vi "add Device.vi"(8 "error in (no error)":errorcluster caption="Fehler (Eingang, kein Fehler)", 10 "Device.lvclass":refnum<class "Device.lvclass">, 11 "Setup Eingang":refnum<class "Setup.lvclass"> caption="DNL_LabVIEW Object in") -> (0 "error out":errorcluster caption="Fehler (Ausgang)", 3 "Setup Ausgang":refnum<class "Setup.lvclass"> caption="DNL_LabVIEW Object out")   [LabVIEW 2013, in "DatenKlassen.lvlib" / "Setup.lvclass"]
uses:
  Setup.lvclass
  Device/Device.lvclass
  Setup.lvclass/Setup.ctl
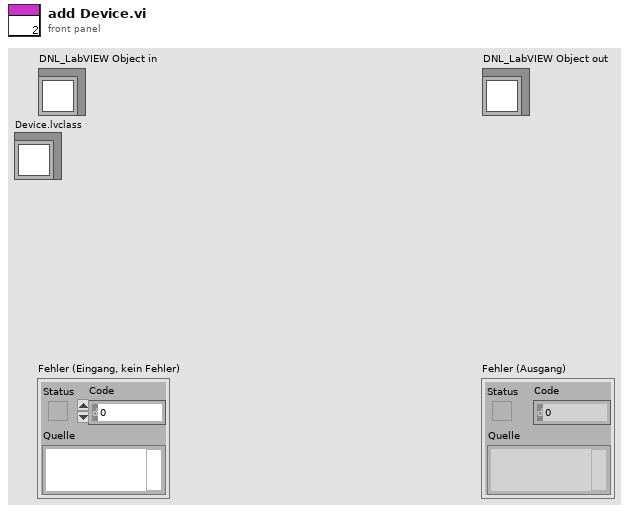
[diagram p1: front panel]
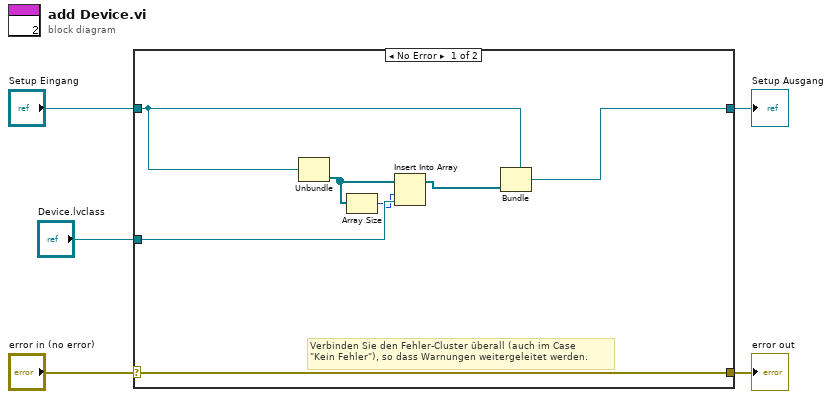
[diagram p0: block diagram]
diagram:
  n1 = case shown="No Error" "error in (no error)" {
    selector: "error in (no error)" -> [w12 w14]
    tunnel: [w12 w14] -> w4
    tunnel: [w11 w13] -> w2
    tunnel: "Setup Eingang" -> [w10 w13]
    tunnel: "Device.lvclass" -> [w9 _]
    frame No Error {
      # "Verbinden Sie den Fehler-Cluster überall (auch im Case\n\"Kein Fehler\"), so dass Warnungen weitergeleitet werden."
      n2 = Unbundle(w10) -> (w6:refnum<class "Device.lvclass">[])  [unwired: 2 out]
      n3 = Array Size(array=w6) -> (size(s)=w7:i32)
      n4 = Insert Into Array(array=w6, index=w7, new element=w9) -> (w8:refnum<class "Device.lvclass">[])
      n5 = Bundle(cluster=w10, w8) -> (w11:refnum<class "Setup.lvclass">)  [unwired: 2 in]
    }
    frame Error {
    }
  }
  "error out" <- w4
  "Setup Ausgang" <- w2
